vi "test16-UserLog_Event.vi"(8 "error in (no error)":errorcluster, 11 "TestCase in":refnum<class "testcase-CSMGlobalLog.lvclass">) -> (0 "error out":errorcluster, 3 "TestCase out":refnum<class "testcase-CSMGlobalLog.lvclass">)   [LabVIEW 2017, in "testcase-CSMGlobalLog.lvclass"]
uses:
  testcase-CSMGlobalLog.lvclass
  testcase-CSMGlobalLog.lvclass/testcase-CSMGlobalLog.ctl
  src/user.lib/_NEVSTOP/Communicable State Machine(CSM)/_Support/Typedef/_CSM_GlobalLog_MSG.ctl
  src/user.lib/_NEVSTOP/Communicable State Machine(CSM)/_Support/Typedef/_CSM_Response Source Message.ctl
  src/user.lib/_NEVSTOP/Communicable State Machine(CSM)/_Support/Typedef/_CSM_GlobalLog_MSG_TYPE.ctl
  c0dc643a-0362-49fc-99f4-5251266ba5a0.vi
  src/user.lib/_NEVSTOP/Communicable State Machine(CSM)/_Support/GlobalEvent/GEvt-Generate with Rule Check.vi
  src/user.lib/_NEVSTOP/Communicable State Machine(CSM)/AdvanceAPI/CSM - Convert Error to Argument.vi
  src/user.lib/_NEVSTOP/Communicable State Machine(CSM)/AdvanceAPI/CSM - Make String Arguments Safe.vi
  src/user.lib/_NEVSTOP/Communicable State Machine(CSM)/AdvanceAPI/CSM - Keywords.vi
  src/user.lib/_NEVSTOP/Communicable State Machine(CSM)/_Support/GlobalEvent/Cache-GEvt Refs.vi
  src/user.lib/_NEVSTOP/Communicable State Machine(CSM)/_Support/GlobalEvent/LogFilter/LogFilter - Check.vi
  src/user.lib/_NEVSTOP/Communicable State Machine(CSM)/_Support/GlobalEvent/LogFilter/LogFilter.lvclass
  <vilib>/addons/_JKI Toolkits/VI Tester/TestCase.llb/TestCase.lvclass
  src/user.lib/_NEVSTOP/Communicable State Machine(CSM)/Communicable State Machine.lvlib
  CSM/CSM-Testcase.lvlib
  C:/Program Files (x86)/National Instruments/LabVIEW 2017/vi.lib/addons/_JKI Toolkits/VI Tester/TestCase.llb/TestCase.lvclass
panel:
  out "String cache each loop":string
  out "LoopCount":i32
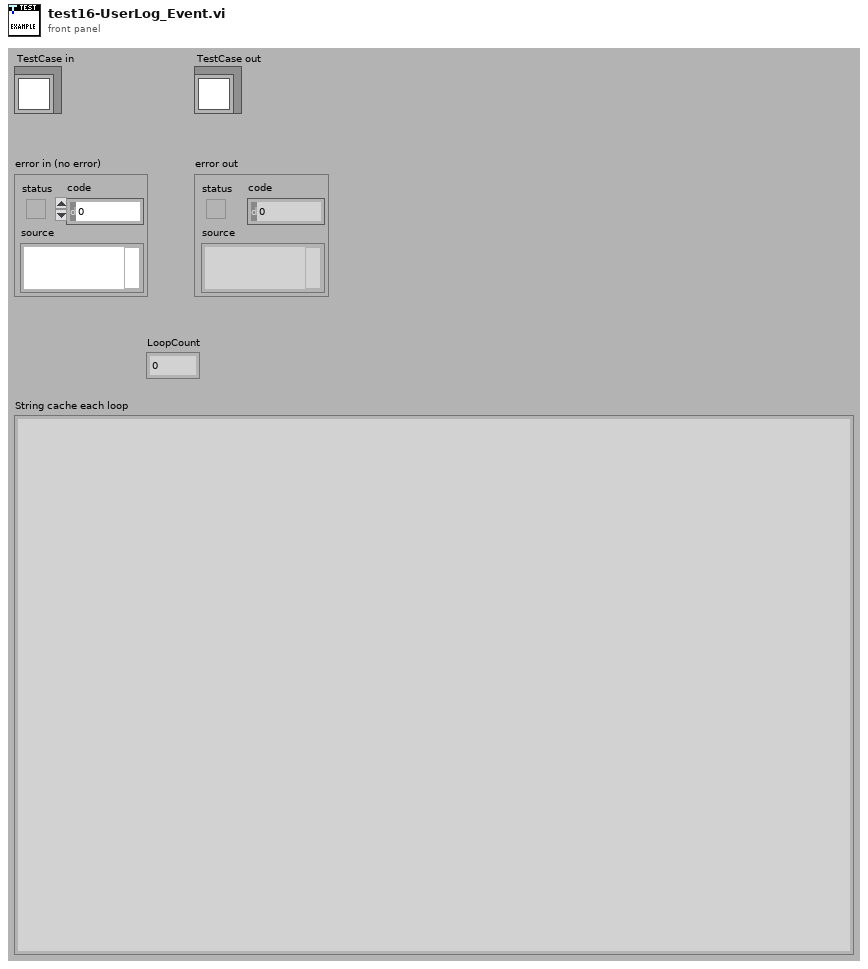
[diagram p1: front panel]
types:
  T1 = typedef "Communicable State Machine.lvlib/_CSM_GlobalLog_MSG.ctl" = cluster{"Name (\"\" to Use UUID)":string, "Current State":string, "Arguments":string, "Source Message":T2, "Source Module":string, "Complete(T)/Start(F)":bool, "LogType":T3, "Time Stamp":timestamp}
  T2 = typedef "Communicable State Machine.lvlib/_CSM_Response Source Message.ctl" = cluster{"‘State":string, "’Arguments":string, "’Error":errorcluster}
  T3 = typedef "Communicable State Machine.lvlib/_CSM_GlobalLog_MSG_TYPE.ctl" = enum16{"User Log", "State Change", "Status", "Interrupt", "Register", "Unregister", "Error Log", "Module Created", "Module Destroyed", "Async Message", "No-Rep Async Message", "Sync Message"}
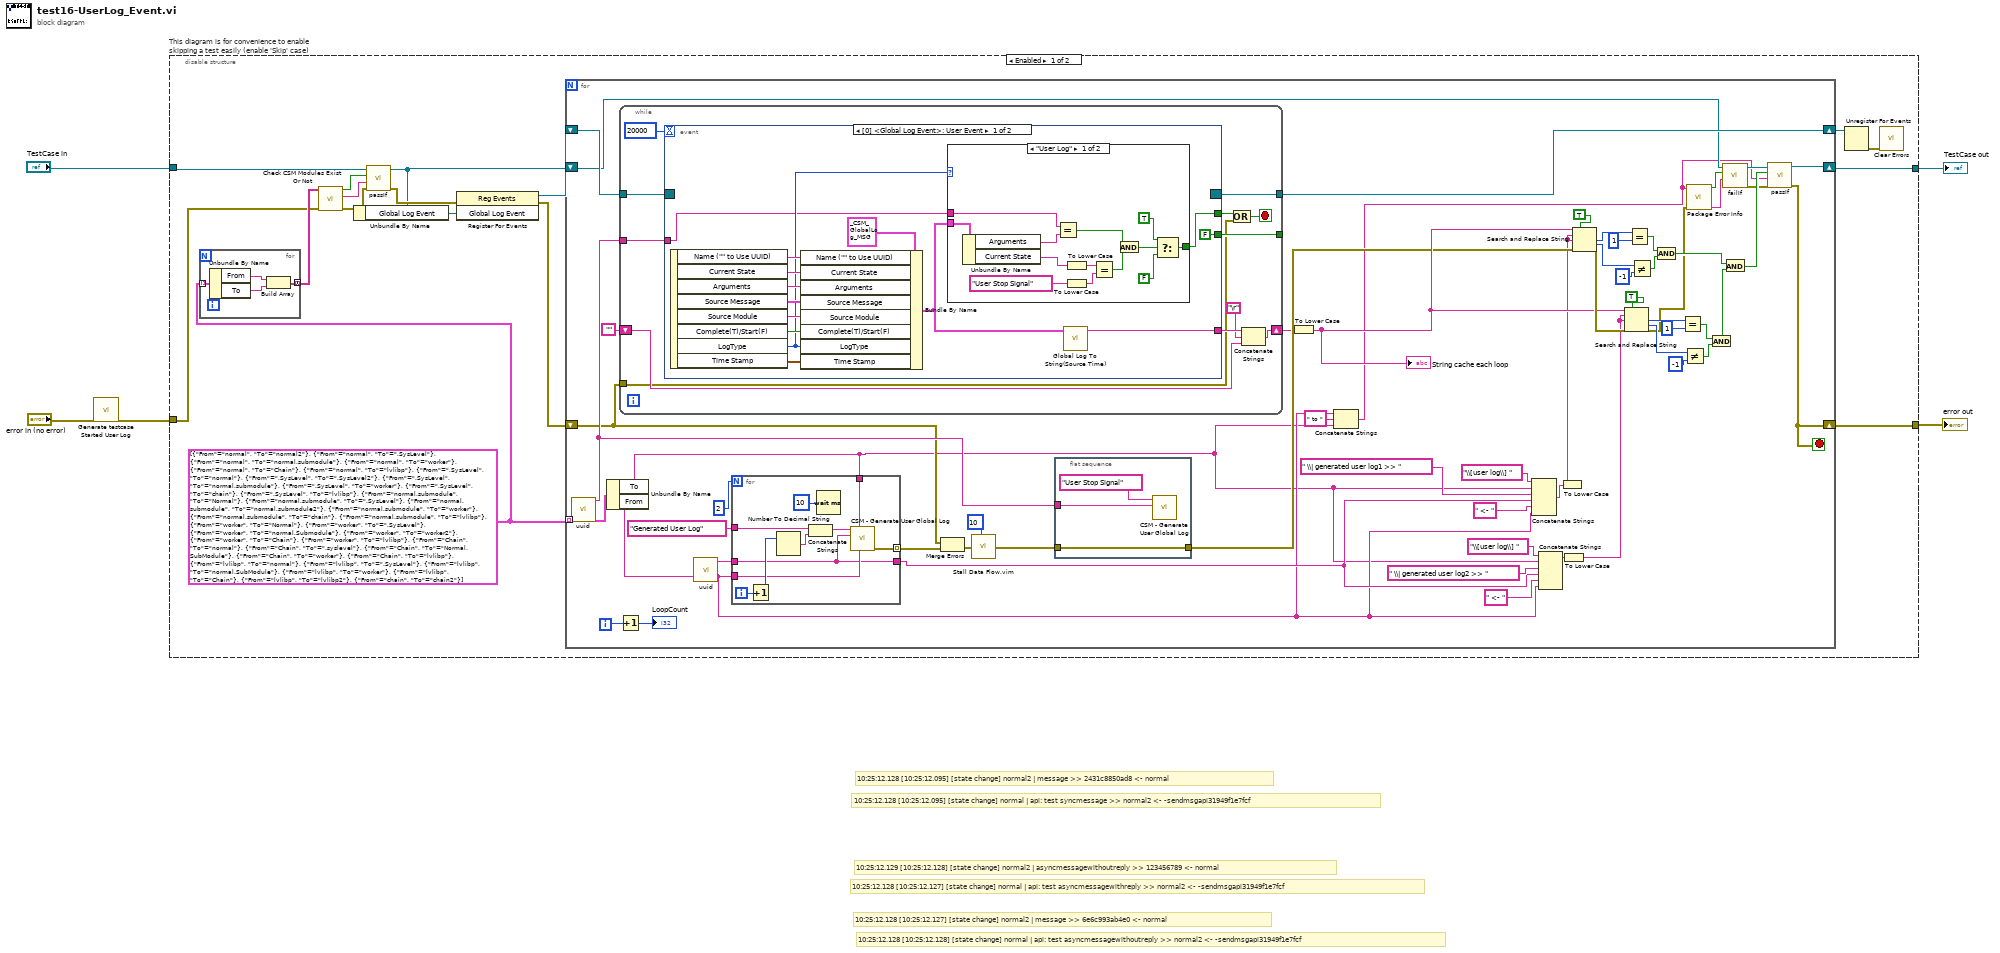
[diagram p0: block diagram]
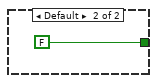
[diagram p2: hidden frame]
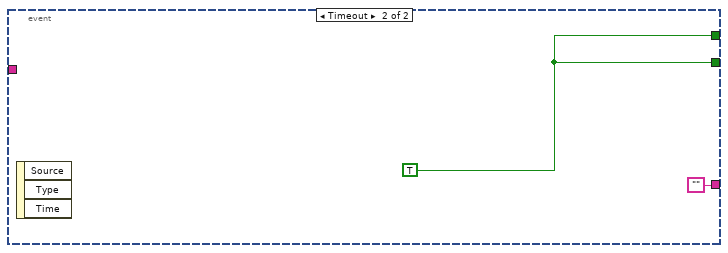
[diagram p3: hidden frame]
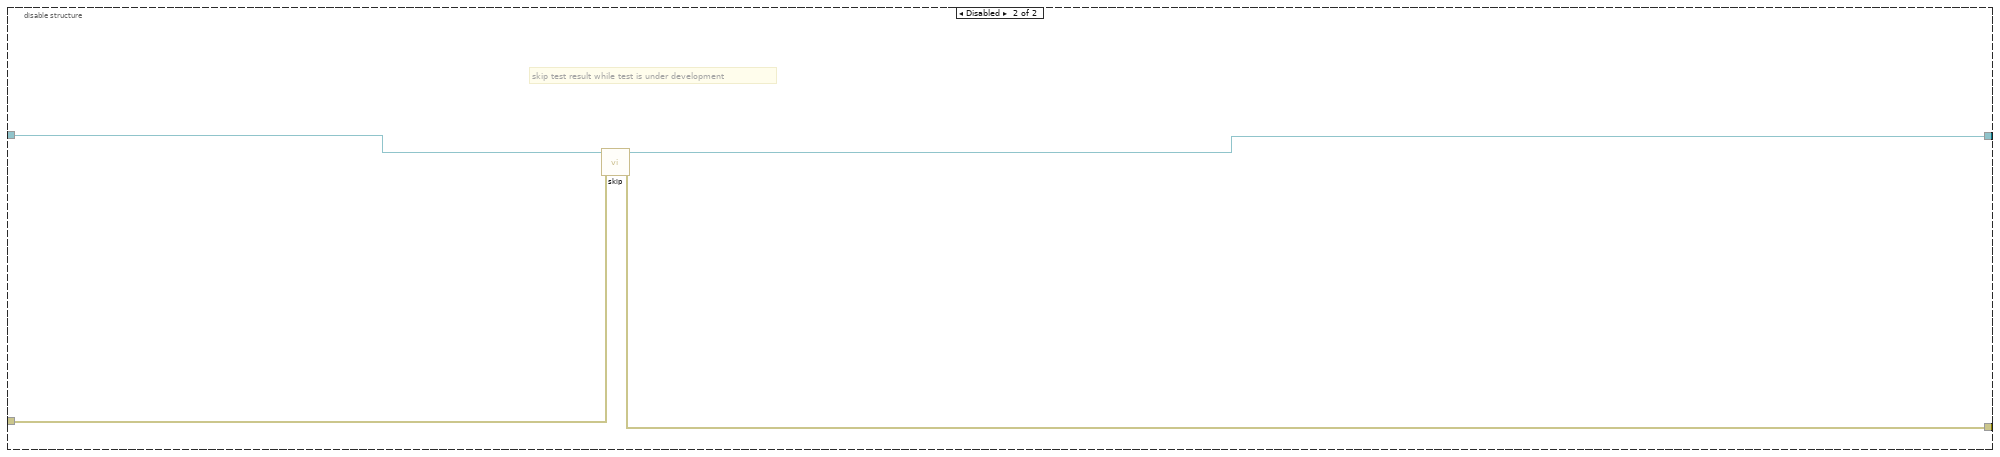
[diagram p4: hidden frame]
diagram:
  # "10:25:12.129 [10:25:12.128] [state change] normal2 | asyncmessagewithoutreply >> 123456789 <- normal"
  # "10:25:12.128 [10:25:12.127] [state change] normal | api: test asyncmessagewithreply >> normal2 <- -sendmsgapi31949f1e7fcf"
  # "10:25:12.128 [10:25:12.127] [state change] normal2 | message >> 6e6c993ab4e0 <- normal"
  # "10:25:12.128 [10:25:12.128] [state change] normal | api: test asyncmessagewithoutreply >> normal2 <- -sendmsgapi31949f1e7fcf"
  # "10:25:12.128 [10:25:12.095] [state change] normal2 | message >> 2431c8850ad8 <- normal"
  # "10:25:12.128 [10:25:12.095] [state change] normal | api: test syncmessage >> normal2 <- -sendmsgapi31949f1e7fcf"
  n1 = call "Generate testcase Started User Log.vi"("Error In"="error in (no error)") -> ("error out"=w1:errorcluster)  [unwired: 10 in]
  n2 = disable-structure "This diagram is for convenience to enable skipping a test easily (enable 'Skip' case)" shown="Enabled" {
    disable-tunnel: "TestCase in" -> [w10 w143]
    disable-tunnel: [w20 w141] -> w2
    disable-tunnel: [w19 w142] -> w4
    disable-tunnel: w1 -> [w11 w140]
    frame Enabled {
      w12 = cluster{"From":string, "To":string}[] [{"From"="normal", "To"="normal2"}, {"From"="normal", "To"=".SysLevel"}, {"From"="normal", "To"="normal.submodule"}, {"From"="normal", "To"="worker"}, {"From"="normal", "To"="Chain"}, {"From"="normal", "To"="lvlibp"}, {"From"=".SysLevel", "To"="normal"}, {"From"=".SysLevel", "To"=".SysLevel2"}, {"From"=".SysLevel", "To"="normal.submodule"}, {"From"=".SysLevel", "To"="worker"}, {"From"=".SysLevel", "To"="chain"}, {"From"=".SysLevel", "To"="lvlibp"}, {"From"="normal.submodule", "To"="Normal"}, {"From"="normal.submodule", "To"=".SysLevel"}, {"From"="normal.submodule", "To"="normal.submodule2"}, {"From"="normal.submodule", "To"="worker"}, {"From"="normal.submodule", "To"="chain"}, {"From"="normal.submodule", "To"="lvlibp"}, {"From"="worker", "To"="Normal"}, {"From"="worker", "To"=".SysLevel"}, {"From"="worker", "To"="normal.Submodule"}, {"From"="worker", "To"="worker2"}, {"From"="worker", "To"="Chain"}, {"From"="worker", "To"="lvlibp"}, {"From"="Chain", "To"="normal"}, {"From"="Chain", "To"=".syslevel"}, {"From"="Chain", "To"="Normal.SubModule"}, {"From"="Chain", "To"="worker"}, {"From"="Chain", "To"="lvlibp"}, {"From"="lvlibp", "To"="normal"}, {"From"="lvlibp", "To"=".SysLevel"}, {"From"="lvlibp", "To"="normal.SubModule"}, {"From"="lvlibp", "To"="worker"}, {"From"="lvlibp", "To"="Chain"}, {"From"="lvlibp", "To"="lvlibp2"}, {"From"="chain", "To"="chain2"}]
      n3 = for {
        tunnel: w12 -> [w25] mode=indexing
        tunnel: [w22] -> w16 mode=concatenating
        n4 = Unbundle By Name(w25) -> ("From"=w24:string, "To"=w23:string)
        n5 = Build Array(w24, w23) -> (w22:string[])
      }
      n6 = call "Check CSM Modules Exist Or Not.vi"("error in"=w11, "CSM names in"=w16) -> ("error out"=w14:errorcluster, "Debug string"=w15:string, "All Modules Exist?"=w17:bool)  [unwired: 7 in]
      n7 = call-dynamic "passIf.vi"("error in (no error)"=w14, "message (\"\")"=w15, "pass"=w17, "TestCase in"=w10) -> ("error out"=w13:errorcluster, "TestCase out"=w9:refnum<class "testcase-CSMGlobalLog.lvclass">)  [unwired: 6 in]
      n8 = Unbundle By Name(w9) -> ("Global Log Event"=w18:refnum<user-event>)
      n9 = register-events(error in=w13, w18) -> (reference out=w7:refnum<event-registration>, error out=w8:errorcluster)  [unwired: 1 in]
      n10 = for {
        shift-right: [w83] -> w21
        shift-left: w7 -> [w84]
        shift-right: [w80] -> w19
        shift-left: w8 -> [w36]
        tunnel: w12 -> [w61] mode=indexing
        shift-right: [w82] -> w20
        shift-left: w9 -> [w33]
        i -> [w58]
        stop <- w80 stop-if-true
        n11 = call "uuid.vi"() -> ("UUID"=w59:string)  [unwired: 11 in]
        n12 = Unbundle By Name(w61) -> ("To"=w28:string, "From"=w29:string)
        n13 = Increment(x=w58) -> (x+1=→"LoopCount":i32)
        n14 = while {
          tunnel: w84 -> [w109]
          tunnel: [w108] -> w83
          shift-right: [w101] -> w53
          shift-left: "" -> [w104]
          tunnel: w59 -> [w106]
          tunnel: [w105] -> _
          tunnel: w36 -> [w98]
          stop <- w100 stop-if-true
          n15 = event shown="[0] <Global Log Event>: User Event" {
            selector: w109 -> [_ _]
            dyn-events: [_ _] -> w108
            timeout: 20000 -> [_ _]
            tunnel: [w110 ""] -> w103
            tunnel: [w112 w139] -> w99
            tunnel: w106 -> [w113 _]
            tunnel: [FALSE ("Stop") w139] -> w105
            event User Event {
              n16 = event-data() -> ("Name (\"\" to Use UUID)"=w122:string, "Current State"=w121:string, "Arguments"=w120:string, "Source Message"=w119:T2, "Source Module"=w118:string, "Complete(T)/Start(F)"=w117:bool, "LogType"=w114:T3, "Time Stamp"=w116:timestamp)  [unwired: 1 in]
              n17 = Bundle By Name(cluster=T1 {"Name (\"\" to Use UUID)"="", "Current State"="", "Arguments"="", "Source Message"={"‘State"="", "’Arguments"="", "’Error"={"status"=FALSE, "code"=0, "source"=""}}, "Source Module"="", "Complete(T)/Start(F)"=FALSE, "LogType"=enum."State Change", "Time Stamp"=timestamp(0 s since 1904-01-01)} ("Cross CSM Data"), "Name (\"\" to Use UUID)"=w122, "Current State"=w121, "Arguments"=w120, "Source Message"=w119, "Source Module"=w118, "Complete(T)/Start(F)"=w117, "LogType"=w114, "Time Stamp"=w116) -> (w111:T1)
              n18 = case shown="\"User Log\"" w114 {
                tunnel: w111 -> [w136 _]
                tunnel: w113 -> [w135 _]
                tunnel: [w124 FALSE] -> w112
                frame "User Log" {
                  n19 = Unbundle By Name(w136) -> ("Arguments"=w134:string, "Current State"=w133:string)
                  n20 = Equal?(x=w135, y=w134) -> (x = y?=w128:bool)
                  n21 = To Lower Case(string=w133) -> (all lower case string=w132:string)
                  n22 = To Lower Case(string="User Stop Signal" ("Log")) -> (all lower case string=w130:string)
                  n23 = Equal?(x=w132, y=w130) -> (x = y?=w129:bool)
                  n24 = And(x=w128, y=w129) -> (x .and. y?=w127:bool)
                  n25 = Select(t=TRUE, s=w127, f=FALSE) -> (s? t:f=w124:bool)
                }
                frame Default {
                }
              }
              n26 = call "Global Log To String(Source Time).vi"("Log"=w111) -> ("Log String"=w110:string)  [unwired: 9 in]
            }
            event Timeout {
              w139 = TRUE ("Stop")
              n27 = event-data() -> ()  [unwired: 1 in, 3 out]
            }
          }
          n28 = Or(x=w99, y=w98) -> (x .or. y?=w100:bool)
          n29 = Concatenate Strings(w103, "\r", w104) -> (w101:string)
        }
        n30 = call "uuid.vi"() -> ("UUID"=w50:string)  [unwired: 11 in]
        n31 = for {
          N: 2 -> [_]
          tunnel: [w94] -> w49 mode=indexing
          tunnel: "Generated User Log" ("Log") -> [w93]
          tunnel: w50 -> [w86]
          tunnel: w28 -> [w88]
          tunnel: w29 -> [w87]
          tunnel: [w86] -> w37
          i -> [w90]
          n32 = Increment(x=w90) -> (x+1=w89:i32)
          n33 = Number To Decimal String(number=w89) -> (decimal integer string=w92:string)  [unwired: 1 in]
          n34 = Concatenate Strings(w93, w92) -> (w91:string)
          n35 = Wait (ms)(milliseconds to wait=u32 10) -> ()  [unwired: 1 out]
          n36 = call "CSM - Generate User Global Log.vi"("From Who"=w87, "Place (\"\" to Use VI's Name)"=w88, "Arguments"=w86, "Log"=w91) -> ("error out"=w94:errorcluster)  [unwired: 7 in]
        }
        n37 = Merge Errors(w36, w49) -> (w48:errorcluster)
        n38 = call "Stall Data Flow.vim"("value in"=w48, "milliseconds to wait"=u32 10) -> ("value out"=w60:errorcluster)  [unwired: 1 out]
        n39 = flat-sequence {
          tunnel: w59 -> [w96]
          tunnel: w60 -> [w95]
          tunnel: [w95] -> w54
          frame #0 {
            n40 = call "CSM - Generate User Global Log.vi"("Arguments"=w96, "Log"="User Stop Signal") -> ()  [unwired: 9 in, 1 out]
          }
        }
        n41 = To Lower Case(string=w53) -> (all lower case string=w55:string)
        "String cache each loop" <- w55
        n42 = Concatenate Strings(w29, " to " ("string"), w28) -> (w26:string)
        n43 = Concatenate Strings("\\[user log\\] " ("regular expression"), w28, " \\| generated user log1 >> " ("string"), w37, " <- " ("string"), w29) -> (w44:string)
        n44 = Concatenate Strings("\\[user log\\] " ("regular expression"), w28, " \\| generated user log2 >> " ("string"), w37, " <- " ("string"), w29) -> (w46:string)
        n45 = To Lower Case(string=w44) -> (all lower case string=w39:string)
        n46 = To Lower Case(string=w46) -> (all lower case string=w38:string)
        n47 = Search and Replace String(replace all?=TRUE ("replace all? (F)"), input string=w55, search string=w39, replace string=w39, error in=w54) -> (number of replacements=w69:i32, offset past replacement=w70:i32, error out=w77:errorcluster)  [unwired: 3 in, 1 out]
        n48 = Search and Replace String(replace all?=TRUE ("replace all? (F)"), input string=w55, search string=w38, replace string=w38, error in=w77) -> (number of replacements=w76:i32, offset past replacement=w75:i32, error out=w30:errorcluster)  [unwired: 3 in, 1 out]
        n49 = Equal?(x=w69, y=1) -> (x = y?=w71:bool)
        n50 = Not Equal?(x=w70, y=-1) -> (x != y?=w72:bool)
        n51 = And(x=w71, y=w72) -> (x .and. y?=w79:bool)
        n52 = Equal?(x=w76, y=1) -> (x = y?=w74:bool)
        n53 = Not Equal?(x=w75, y=-1) -> (x != y?=w73:bool)
        n54 = call "Package Error Info.vi"("error in"=w30, "String in"=w26) -> ("packed error info out"=w34:string, "error status"=w35:bool)  [unwired: 8 in]
        n55 = And(x=w74, y=w73) -> (x .and. y?=w78:bool)
        n56 = call-dynamic "failIf.vi"("message (\"\")"=w34, "fail"=w35, "TestCase in"=w33) -> ("error out"=w31:errorcluster, "TestCase out"=w32:refnum<class "testcase-CSMGlobalLog.lvclass">)  [unwired: 7 in]
        n57 = And(x=w79, y=w78) -> (x .and. y?=w57:bool)
        n58 = call-dynamic "passIf.vi"("error in (no error)"=w31, "message (\"\")"=w26, "pass"=w57, "TestCase in"=w32) -> ("error out"=w80:errorcluster, "TestCase out"=w82:refnum<class "testcase-CSMGlobalLog.lvclass">)  [unwired: 6 in]
      }
      n59 = Unregister For Events(event registration refnum=w21) -> (error out=w6:errorcluster)  [unwired: 1 in]
      n60 = call <vilib>:"Clear Errors.vi"("error in (no error)"=w6) -> ()  [unwired: 5 in, 2 out]
    }
    frame Disabled {
      # "skip test result while test is under development"
      n61 = call <vilib>:"skip.vi"("error in (no error)"=w140, "TestCase in"=w143) -> ("error out"=w142:errorcluster, "TestCase out"=w141:refnum<class "testcase-CSMGlobalLog.lvclass">)  [unwired: 8 in]
    }
  }
  "error out" <- w4
  "TestCase out" <- w2
